vi "RyanTesting.vi"() -> ()   [LabVIEW 2016]
panel:
  out "Battery  2":cluster{dbl[], dbl[]}[](graph)
  in  "Boolean 2":bool
  in  "UPPER LIMIT 2":u32=36
  in  "UPPER LIMIT":u32=36
  in  "Boolean":bool
  out "Battery":cluster{dbl[], dbl[]}[](graph)
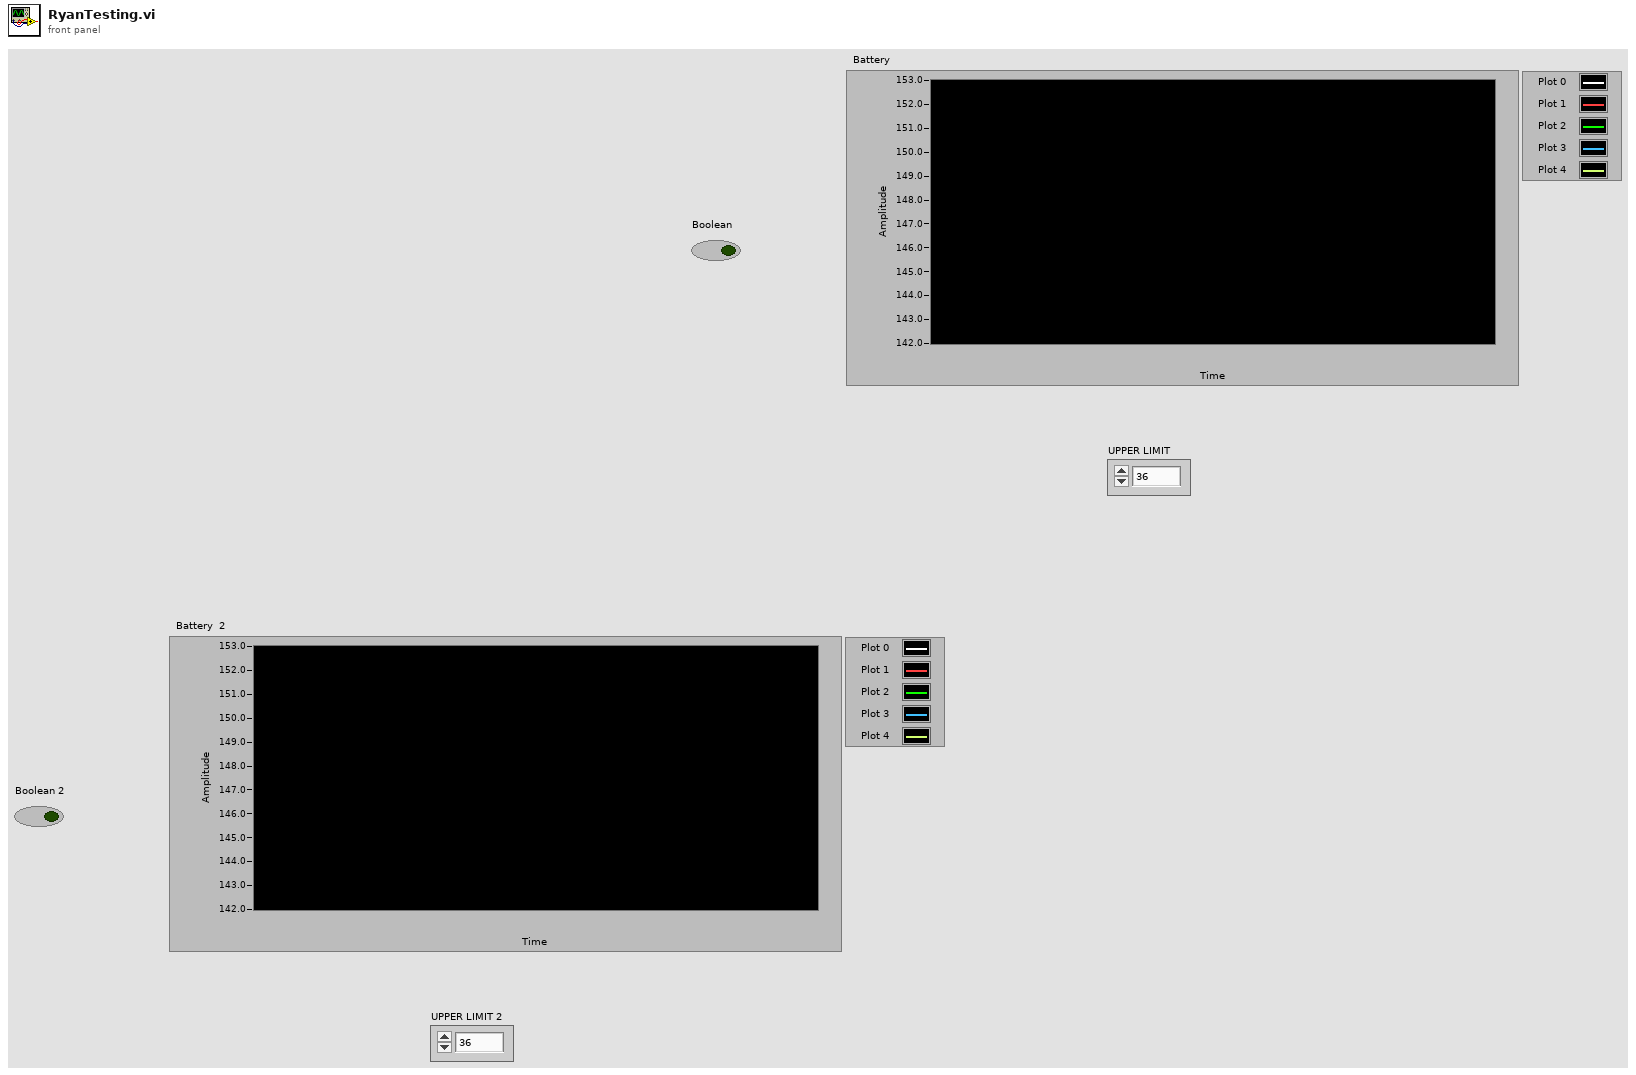
[diagram p1: front panel]
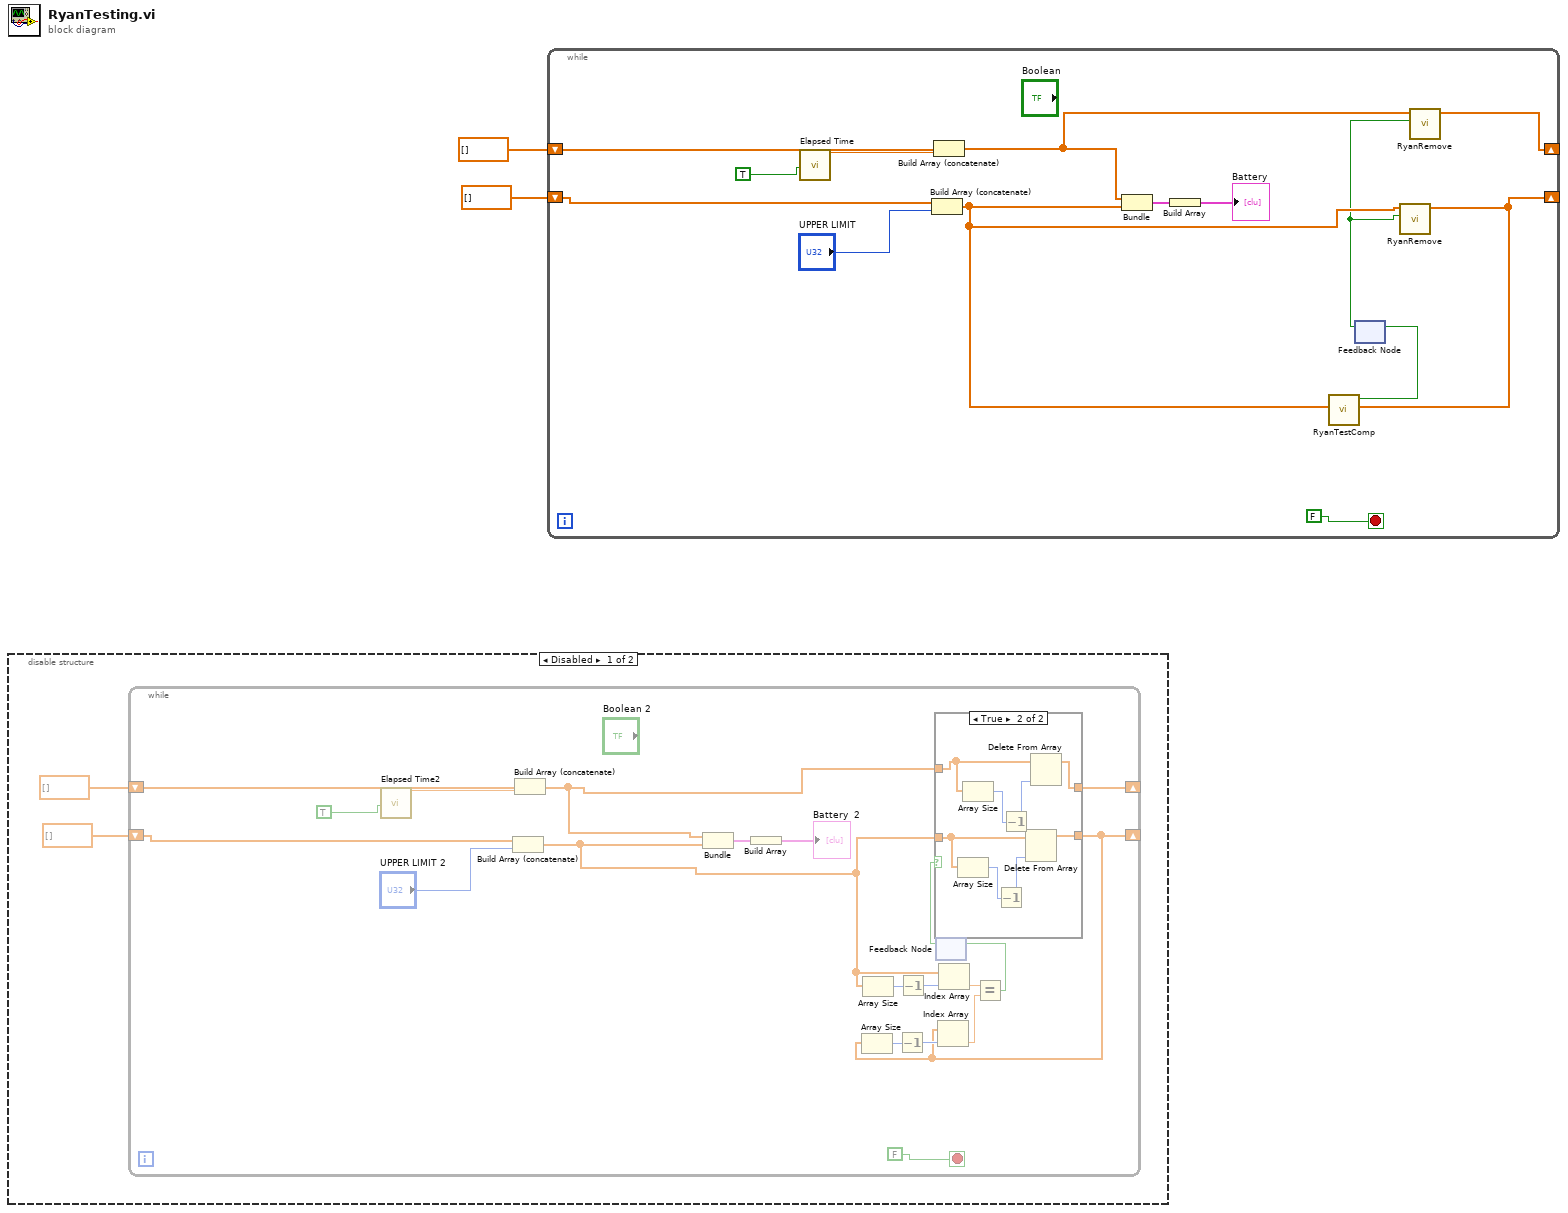
[diagram p0: block diagram]
diagram:
  n1 = disable-structure shown="Disabled" {
    frame Disabled {
      n2 = while {
        shift-right: [w10] -> _
        shift-left: dbl[] [] ("Array") -> [w22]
        shift-right: [w17] -> _
        shift-left: dbl[] [] ("Array") -> [w23]
        stop <- FALSE stop-if-true
        n3 = call "Elapsed Time2"("Auto Reset"=TRUE) -> ("Present (s)"=w24:dbl)  [unwired: 11 in, 7 out]
        n4 = Build Array (concatenate)(w22, "UPPER LIMIT 2") -> (w14:dbl[])
        n5 = Build Array (concatenate)(w23, w24) -> (w19:dbl[])
        n6 = Bundle(w19, w14) -> (w5:cluster{dbl[], dbl[]})  [unwired: 1 in]
        n7 = Build Array(w5) -> (→"Battery  2":cluster{dbl[], dbl[]}[])
        n8 = Array Size(array=w14) -> (size(s)=w16:i32)
        n9 = Decrement(x=w16) -> (x-1=w15:i32)
        n10 = feedback #1() -> (w7:bool)  [unwired: 1 in]
        n11 = case shown="True" w7 {
          tunnel: [w26 w34] -> w10
          tunnel: w14 -> [w26 w32]
          tunnel: w19 -> [w25 w28]
          tunnel: [w25 w27] -> w17
          frame False {
          }
          frame True {
            n12 = Array Size(array=w32) -> (size(s)=w33:i32)
            n13 = Array Size(array=w28) -> (size(s)=w30:i32)
            n14 = Decrement(x=w33) -> (x-1=w31:i32)
            n15 = Decrement(x=w30) -> (x-1=w29:i32)
            n16 = Delete From Array(array=w32, index=w31) -> (array with subset deleted=w34:dbl[])  [unwired: 1 in, 1 out]
            n17 = Delete From Array(array=w28, index=w29) -> (array with subset deleted=w27:dbl[])  [unwired: 1 in, 1 out]
          }
        }
        n18 = Array Size(array=w10) -> (size(s)=w12:i32)
        n19 = Decrement(x=w12) -> (x-1=w11:i32)
        n20 = Index Array(array=w10, index=w11) -> (element=w9:dbl)
        n21 = Index Array(array=w14, index=w15) -> (element=w13:dbl)
        n22 = Equal?(x=w13, y=w9) -> (x = y?=w8:bool)
        n23 = feedback-in #1(w8) -> ()
      }
    }
    frame Enabled {
    }
  }
  n24 = while {
    shift-right: [w36] -> _
    shift-left: dbl[] [] ("Array") -> [w46]
    shift-right: [w41] -> _
    shift-left: dbl[] [] ("Array") -> [w47]
    stop <- FALSE stop-if-true
    n25 = call "Elapsed Time"("Auto Reset"=TRUE) -> ("Present (s)"=w48:dbl)  [unwired: 11 in, 7 out]
    n26 = Build Array (concatenate)(w46, "UPPER LIMIT") -> (w37:dbl[])
    n27 = Build Array (concatenate)(w47, w48) -> (w43:dbl[])
    n28 = Bundle(w43, w37) -> (w38:cluster{dbl[], dbl[]})  [unwired: 1 in]
    n29 = Build Array(w38) -> (→"Battery":cluster{dbl[], dbl[]}[])
    n30 = feedback #2() -> (w35:bool)  [unwired: 1 in]
    n31 = call "RyanRemove.vi"("Boolean"=w35, "IN"=w37) -> ("OUT"=w36:dbl[])  [unwired: 9 in]
    n32 = call "RyanTestComp.vi"("NEW"=w37, "OLD"=w36) -> ("Boolean"=w40:bool)  [unwired: 9 in]
    n33 = feedback-in #2(w40) -> ()
    n34 = call "RyanRemove.vi"("Boolean"=w35, "IN"=w43) -> ("OUT"=w41:dbl[])  [unwired: 9 in]
  }
